vi "Read Abort Notifier.vi"(11 "Job in":refnum<class "Job.lvclass">) -> (2 "Abort":refnum<notifier>)   [LabVIEW 2013, in "openCronJob.lvlib" / "Job.lvclass"]
uses:
  Job.lvclass
  Job.lvclass/Job.ctl
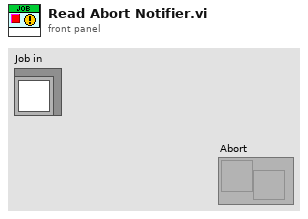
[diagram p1: front panel]
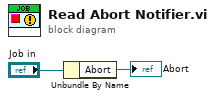
[diagram p0: block diagram]
diagram:
  n1 = Unbundle By Name("Job in") -> ("Abort"=→"Abort":refnum<notifier>)
